vi "RSZVB Edit Ripple Limit Line Segment.vi"(6 "Start Stimulus (0.0)":dbl format="%^.3e", 7 "Stop Stimulus (0.0)":dbl format="%^.3e", 8 "error in (no error)":errorcluster {"code" format="%.0x"}, 9 "Segment (1)":i32=1, 10 "Channel (Trace) (1)":i32=1, 11 "VISA session":refnum<visa-resource-name>) -> (0 "error out":errorcluster {"code" format="%.0x"}, 3 "dup VISA session":refnum<visa-resource-name>)   [LabVIEW 2011]
doc: "This VI edits existing segment of the ripple limit line segments list.\n\nNote(s):\n\n(1) To define several ripple limit ranges with a single command\nuse CALCulate<Chn>:RIPPle\n\nRemote-control command(s):\nCALCulate<Chn>:RIPPle:SEGMent<Seg>:STIMulus:STARt <numeric_value>\nCALCulate<Chn>:RIPPle:SEGMent<Seg>:STIMulus:STOP <numeric_value>"
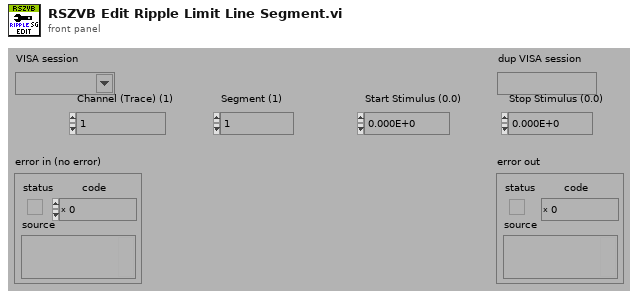
[diagram p1: front panel]
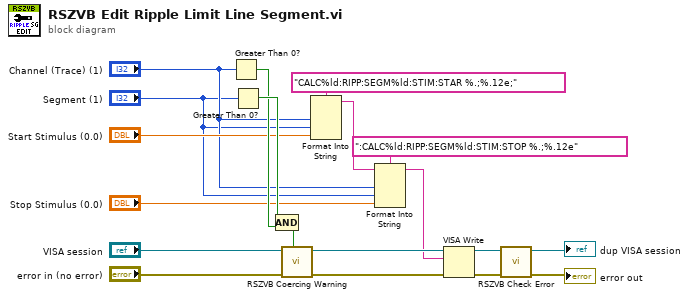
[diagram p0: block diagram]
diagram:
  n1 = Greater Than 0?(x="Channel (Trace) (1)") -> (x > 0?=w12:bool)
  n2 = Greater Than 0?(x="Segment (1)") -> (x > 0?=w13:bool)
  n3 = Compound Arithmetic op=AND(w13, w12) -> (w14:bool)
  n4 = call "RSZVB Coercing Warning.vi"("In Range?"=w14, "error in (no error)"="error in (no error)", "VISA session"="VISA session") -> ("error out"=w17:errorcluster, "dup VISA session"=w18:refnum<visa-resource-name>)  [unwired: 7 in]
  n5 = Format Into String(format string="CALC%ld:RIPP:SEGM%ld:STIM:STAR %.;%.12e;", "Channel (Trace) (1)", "Segment (1)", "Start Stimulus (0.0)") -> (resulting string=w4:string)  [unwired: 2 in, 1 out]
  n6 = Format Into String(format string=":CALC%ld:RIPP:SEGM%ld:STIM:STOP %.;%.12e", initial string=w4, "Channel (Trace) (1)", "Segment (1)", "Stop Stimulus (0.0)") -> (resulting string=w3:string)  [unwired: 1 in, 1 out]
  n7 = VISA Write(VISA resource name=w18, write buffer=w3, error in (no error)=w17) -> (VISA resource name out=w15:refnum<visa-resource-name>, error out=w16:errorcluster)  [unwired: 1 out]
  n8 = call "RSZVB Check Error.vi"("error in (no error)"=w16, "VISA session"=w15) -> ("error out"=→"error out":errorcluster, "dup VISA session"=→"dup VISA session":refnum<visa-resource-name>)  [unwired: 8 in]
